vi "Antipinch.vi"(7 "Model Name":T3, 8 "Error In":errorcluster, 9 "Intialize?":bool=TRUE, 10 "Inputs":T1, 11 "Start SM":dbl=20.0 format="%#_13g") -> (0 "error out":errorcluster, 1 "Completed":bool, 3 "Results":cluster{"Pinch Force":dbl}, 4 "Status":cluster{"Status":string, "Elapsed Time":dbl}, 5 "Graph":dbl[][](array[numeric]))   [LabVIEW 2017]
doc: "Changelog:\n\n------------\nv0.1:\n- Bypass sensor 1 for all front\n\nv0.1:\n- Start Travel time taken from when the start moving command is given (previous state)\n- Total travel time is taken until the movement is stopped"
uses:
  controls/Model Name.ctl
  controls/All Inputs.ctl
  controls/SACB DI.ctl
  controls/Antipinch.ctl
  controls/FGV DO.ctl
panel:
  out "x/y":dbl
  in  "minimum change":dbl=2.0 format="%#_13g"
  in  "AutoCommand":u32=50
  in  "Stall Time":u32=200
  out "Waveform Graph":dbl[][](graph)
  in  "Delay (for Rest)":u32=500
  in  "Timeout (ms)":u32=15000
  # "Inputs"
  # "Variables"
  # "Outputs"
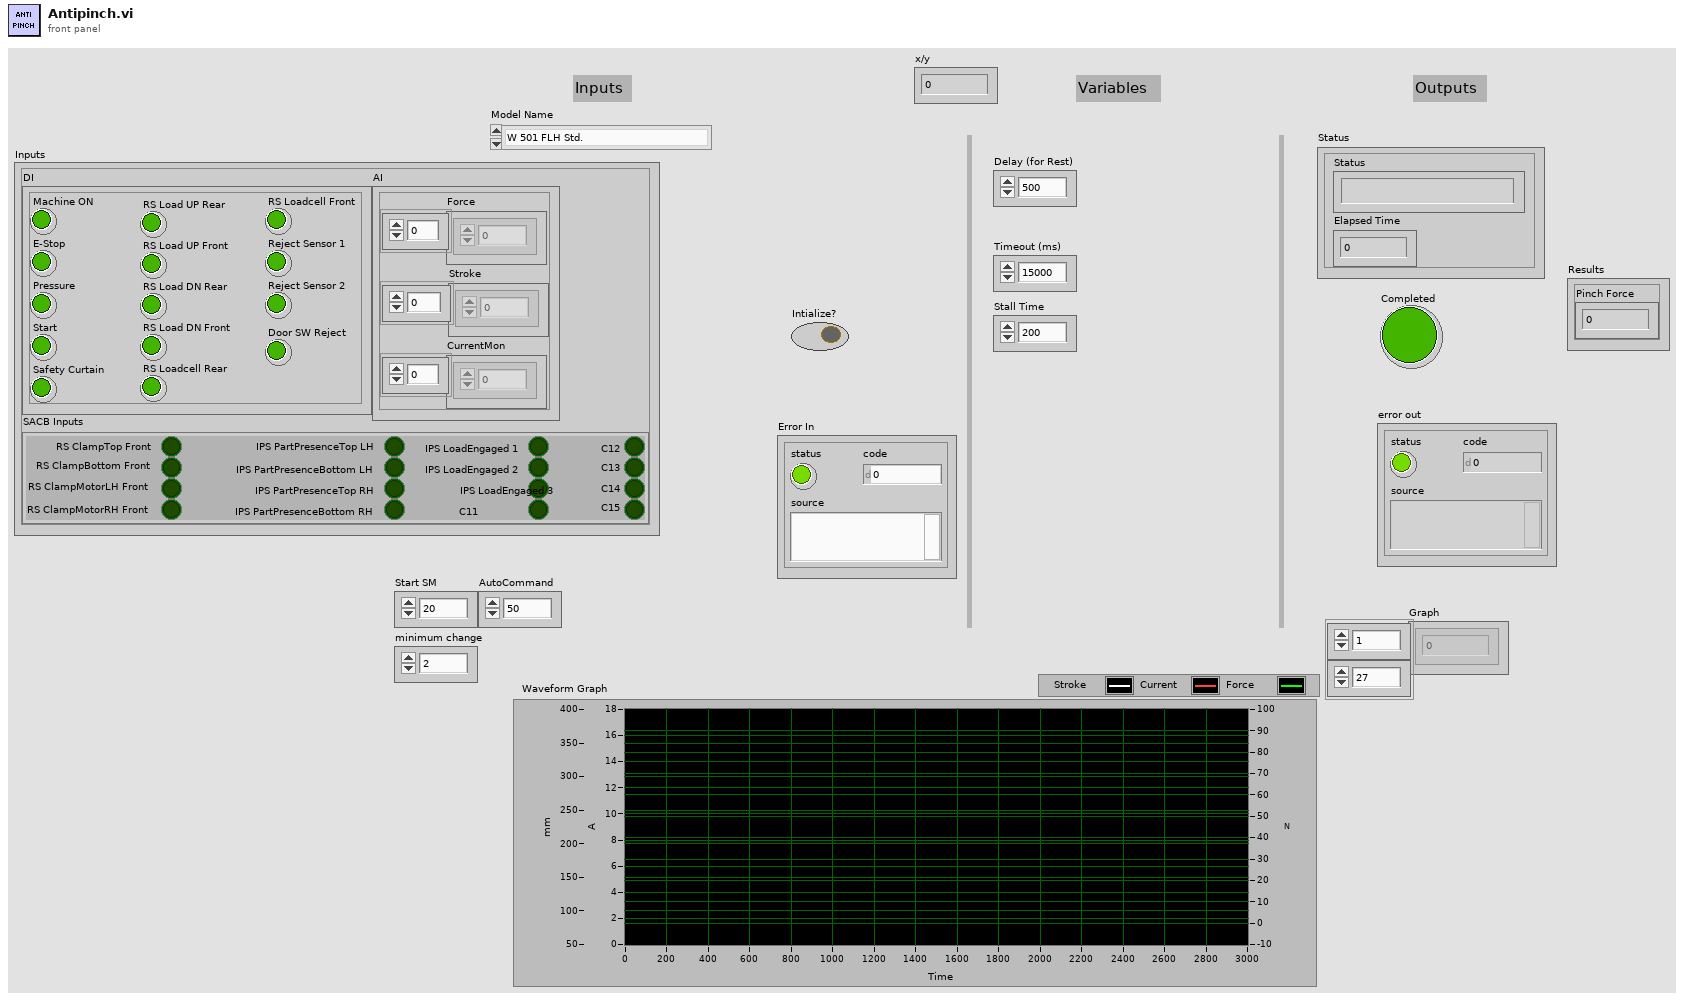
[diagram p1: front panel]
types:
  T1 = typedef "All Inputs.ctl" = cluster{"DI":cluster{"Machine ON":bool, "E-Stop":bool, "Pressure":bool, "Start":bool, "Safety Curtain":bool, "RS Load UP Rear":bool, "RS Load UP Front":bool, "RS Load DN Rear":bool, "RS Load DN Front":bool, "RS Loadcell Rear":bool, "RS Loadcell Front":bool, "Reject Sensor 1":bool, "Reject Sensor 2":bool, "Door SW Reject":bool}, "AI":cluster{"Force":dbl[], "Stroke":dbl[], "CurrentMon":dbl[]}, "SACB Inputs":T2}
  T2 = typedef "SACB DI.ctl" = cluster{"RS ClampTop Front":bool, "RS ClampBottom Front":bool, "RS ClampMotorLH Front":bool, "RS ClampMotorRH Front":bool, "IPS PartPresenceTop LH":bool, "IPS PartPresenceBottom LH":bool, "IPS PartPresenceTop RH":bool, "IPS PartPresenceBottom RH":bool, "IPS LoadEngaged 1":bool, "IPS LoadEngaged 2":bool, "IPS LoadEngaged 3":bool, "C11":bool, "C12":bool, "C13":bool, "C14":bool, "C15":bool}
  T3 = typedef "Model Name.ctl" = enum16{"W 501 FLH Std.", "W 501 FRH Std.", "W 601 FR RH Std", "W 601 FR LH Std", "W 601 RR RH Std", "W 601 RR LH Std", "W 601 FR RH AP", "W 601 FR LH AP", "W 601 RR RH AP", "W 601 RR LH AP"}
  T4 = typedef "Antipinch.ctl" = enum16{"Initialize", "Check Bottom Position", "Auto UP-1", "Auto UP-2", "Loadcell Front", "Wait for Pinch", "Wait for Reversal", "Wait for Stop", "Loadcell Rear & Rest", "Done", "Error"}
  T5 = typedef "FGV DO.ctl" = enum16{"Initialize", "Start Task", "Clamping", "Load CYL", "Contactors", "Loadcell CYL", "BSL", "Read DO", "Clear Tasks", "Clear Task"}
  T6 = typedef "AntiPinch.ctl" = enum16{"Initialize", "Check Bottom Position", "Auto UP-1", "Auto UP-2", "Loadcell Front", "Wait for Pinch", "Wait for Reversal", "Wait for Stop", "Loadcell Rear & Rest", "Done", "Error"}
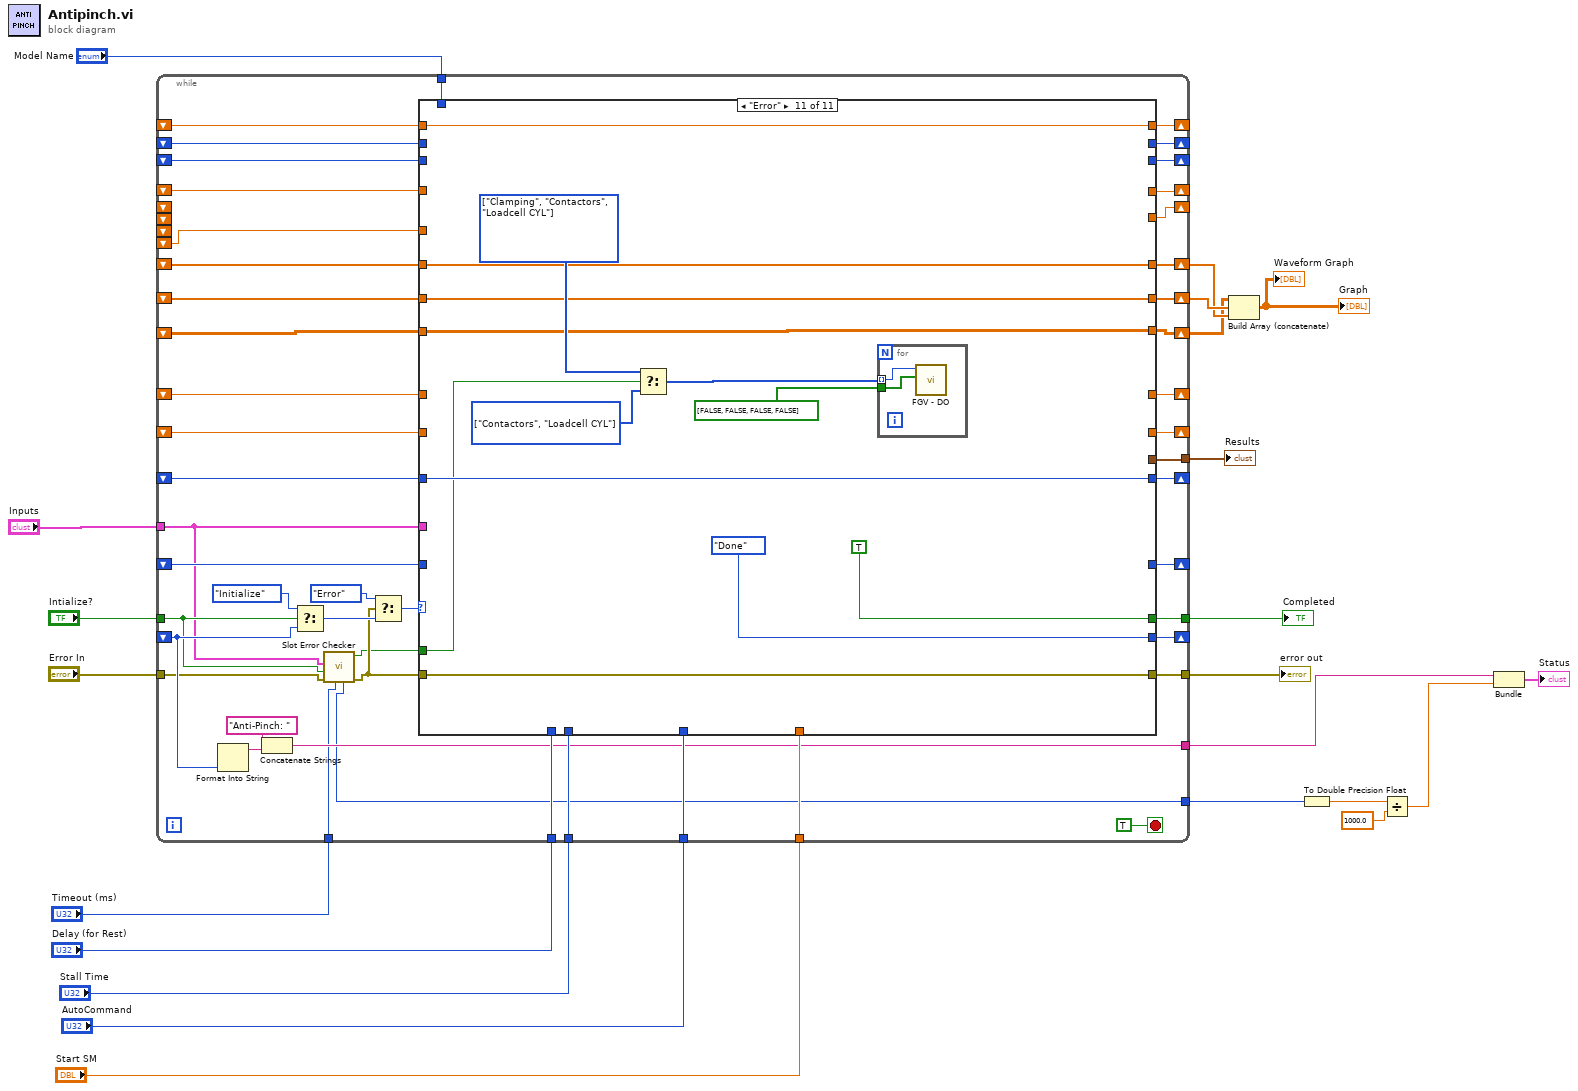
[diagram p0: block diagram]
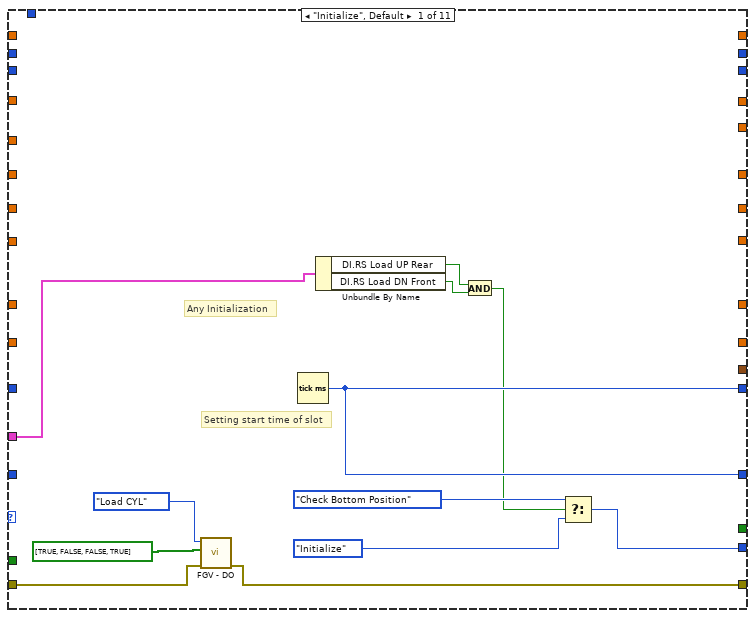
[diagram p2: hidden frame]
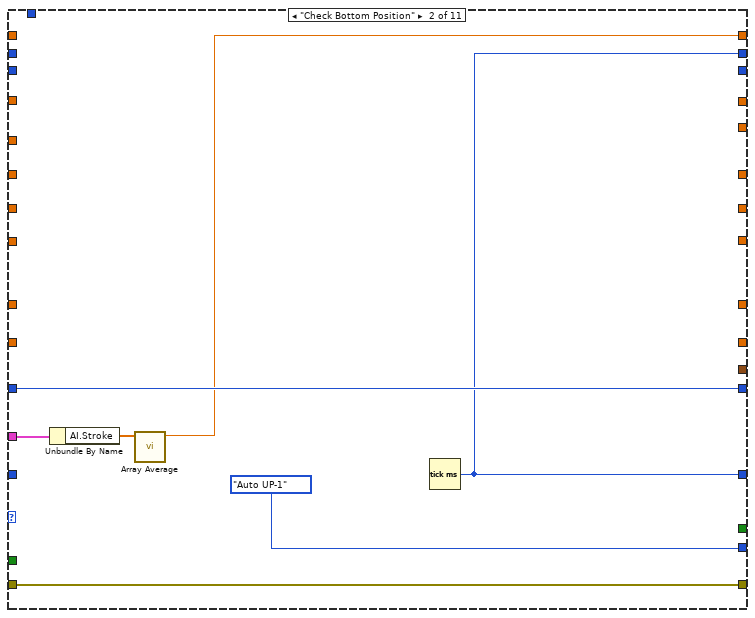
[diagram p3: hidden frame]
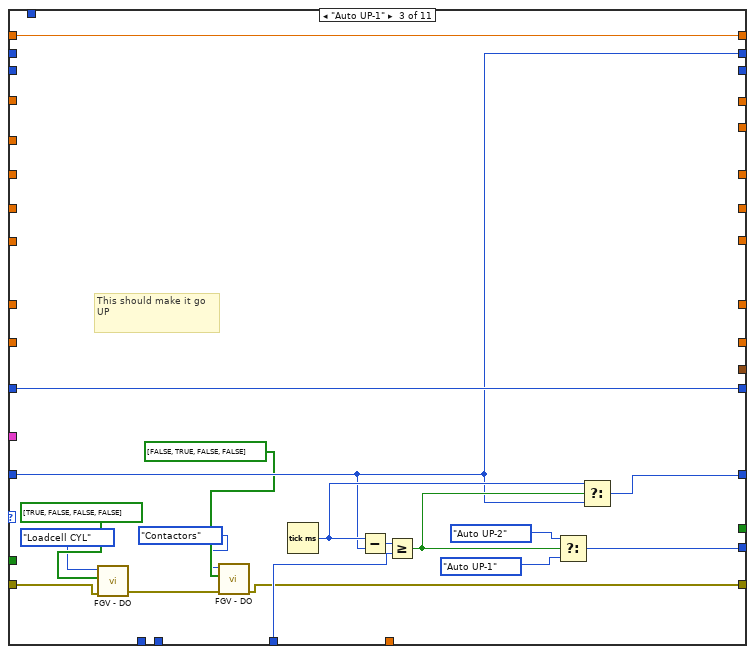
[diagram p4: hidden frame]
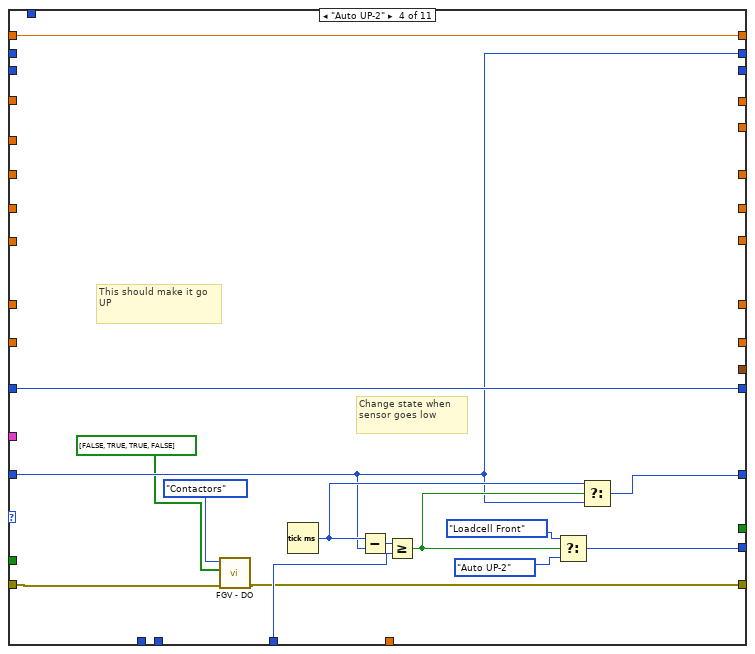
[diagram p5: hidden frame]
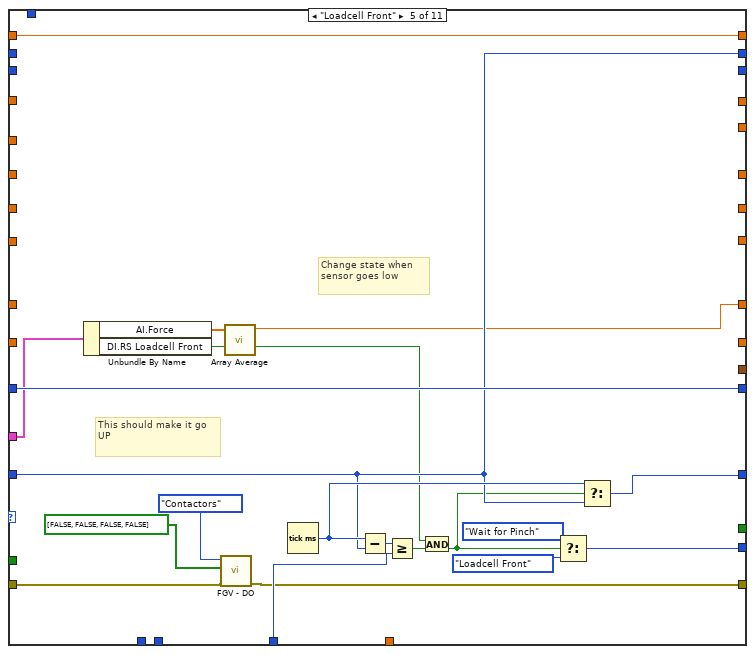
[diagram p6: hidden frame]
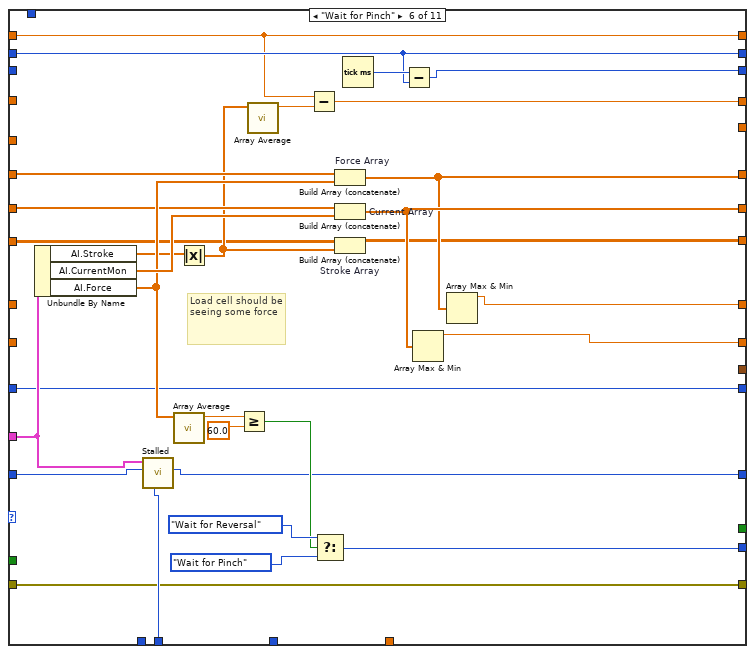
[diagram p7: hidden frame]
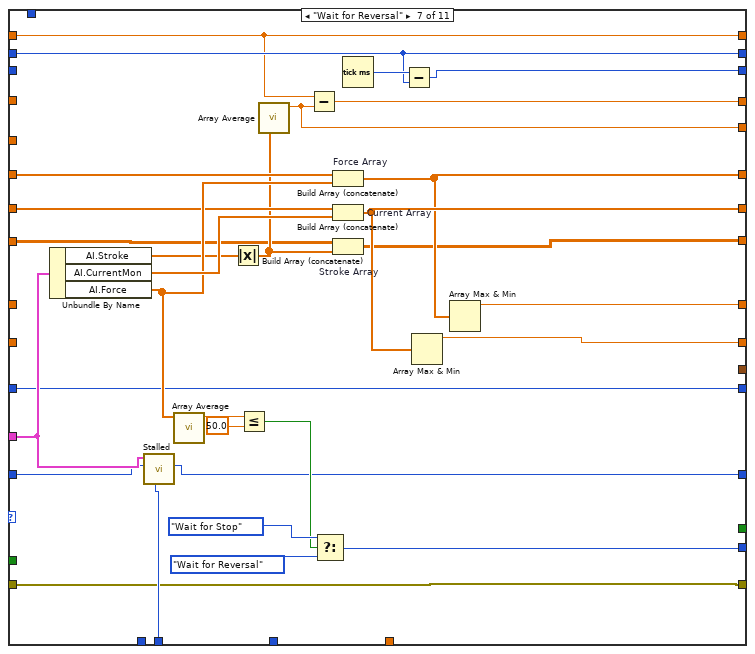
[diagram p8: hidden frame]
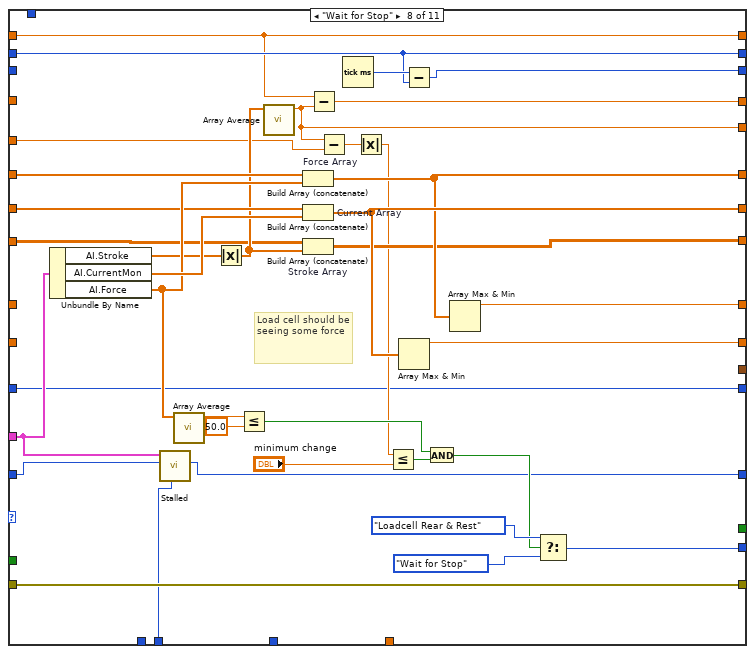
[diagram p9: hidden frame]
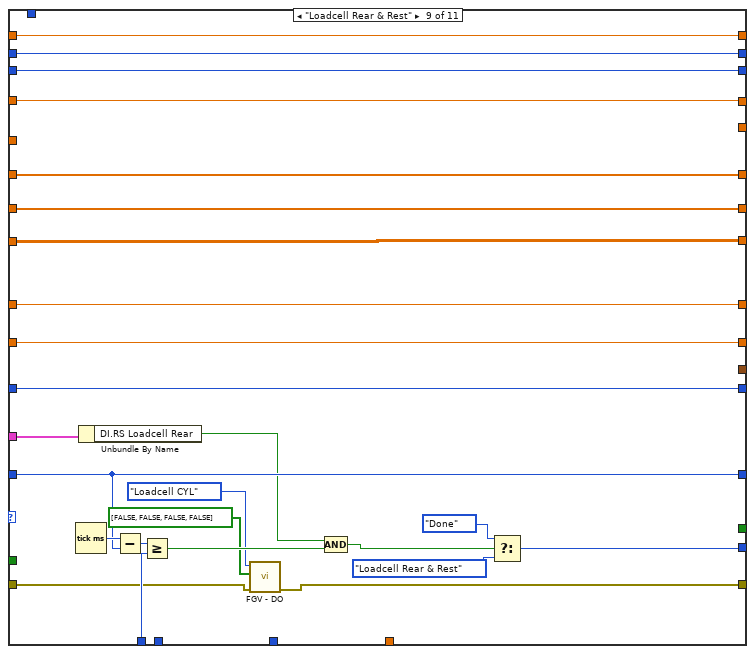
[diagram p10: hidden frame]
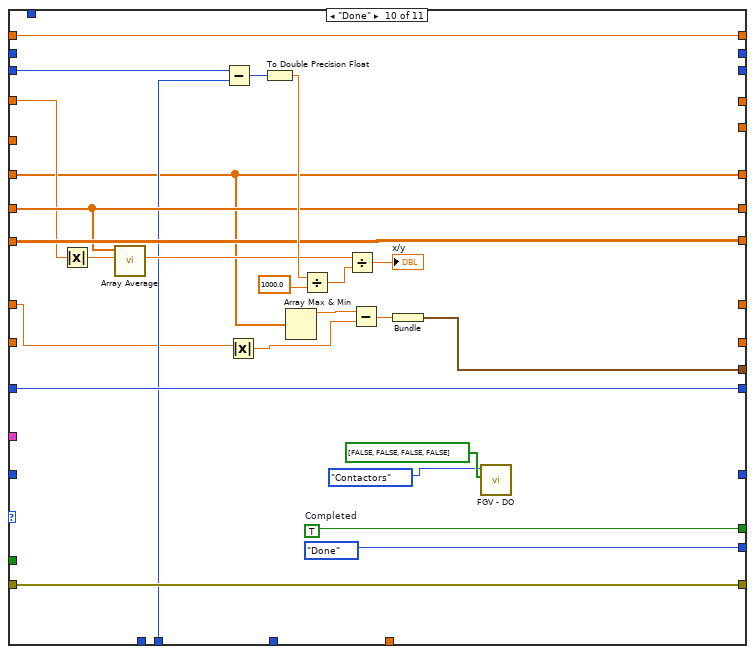
[diagram p11: hidden frame]
diagram:
  n1 = while {
    tunnel: "Intialize?" -> [w30]
    shift-right: [w69] -> _
    shift-left: _ -> [w32]
    shift-right: [w68] -> _
    shift-left: _ -> [w67]
    tunnel: "Error In" -> [w31]
    tunnel: [w66] -> w22
    tunnel: [w65] -> w21
    tunnel: "Inputs" -> [w29]
    tunnel: "Delay (for Rest)" -> [w62]
    tunnel: "Timeout (ms)" -> [w27]
    tunnel: "Model Name" -> [w61]
    shift-right: [w60] -> _
    shift-left: _ -> [w59]
    shift-right: [w58] -> w2
    shift-left: _ -> [w57]
    shift-right: [w56] -> _
    shift-left: _ -> [w55]
    tunnel: [w54] -> w15
    shift-right: [w53] -> _
    shift-left: _ -> [w52]
    tunnel: [w26] -> w10
    shift-right: [w50] -> _
    shift-left: _ -> [w49]
    shift-right: [w48] -> w9
    shift-left: _ -> [w47]
    shift-right: [w46] -> w7
    shift-left: _ -> [w45]
    shift-right: [w44] -> _
    shift-left: _ -> [w43]
    shift-right: [w42] -> _
    shift-left: _ -> [w41]
    tunnel: "Stall Time" -> [w40]
    tunnel: "Start SM" -> [w39]
    tunnel: "AutoCommand" -> [w38]
    shift-right: [w37] -> _
    shift-left: _ -> [_]
    shift-left: _ -> [_]
    shift-left: _ -> [_]
    shift-left: _ -> [w36]
    tunnel: [w33] -> w3
    shift-right: [w24] -> _
    shift-left: _ -> [w23]
    stop <- TRUE stop-if-true
    n2 = Format Into String(w32) -> (resulting string=w35:string)  [unwired: 3 in, 1 out]
    n3 = Concatenate Strings("Anti-Pinch: ", w35) -> (w33:string)
    n4 = Select(t=Antipinch."Initialize", s=w30, f=w32) -> (s? t:f=w64:T4)
    n5 = call "Slot Error Checker.vi"("Timeout (ms)"=w27, "error in (no error)"=w31, "Intialize?"=w30, "Inputs"=w29) -> ("error out"=w28:errorcluster, "Safety Interrupt?"=w25:bool, "Slot Time"=w26:u32)  [unwired: 5 in]
    n6 = Select(t=Antipinch."Error", s=w28, f=w64) -> (s? t:f=w51:T4)
    n7 = case shown="\"Error\"" w51 {
      tunnel: [w81 AntiPinch."Auto UP-1" w104 w119 w139 w171 w201 w237 w261 Antipinch."Done" Antipinch."Done"] -> w69
      tunnel: [w83 w84 w99 w114 w134 w149 w178 w207 w263 _ _] -> w68
      tunnel: w67 -> [_ _ w100 w115 w135 w150 w179 w209 w263 _ _]
      tunnel: w28 -> [w73 w89 w96 w110 w125 w146 w175 w220 w241 w287 w301]
      tunnel: [w72 w89 w92 w109 w124 w146 w175 w220 w240 w287 w301] -> w66
      tunnel: [_ _ _ _ _ _ _ _ _ w286 TRUE ("Completed")] -> w65
      tunnel: w29 -> [w79 w86 _ _ w132 w145 w180 w205 w244 _ _]
      tunnel: [w83 w90 w108 w123 w143 w144 w174 w204 w257 w285 w298] -> w24
      tunnel: w23 -> [_ w90 w108 w123 w143 w144 w174 w204 w257 w285 w298]
      tunnel: w62 -> [_ _ _ _ _ _ _ _ w256 _ _]
      tunnel: w61 -> [_ _ _ _ _ _ _ _ _ _ _]
      tunnel: [_ w84 w100 w115 w135 w163 w193 w229 w253 _ _] -> w60
      tunnel: w59 -> [_ _ _ _ _ w163 w193 w229 w253 _ _]
      tunnel: [_ _ _ _ _ w164 w194 w230 w255 w280 w291] -> w58
      tunnel: w57 -> [_ _ _ _ _ w151 w181 w210 w255 w280 w291]
      tunnel: [_ _ _ _ _ w165 w195 w231 w254 _ _] -> w56
      tunnel: w55 -> [_ _ _ _ _ _ _ _ w254 w276 _]
      tunnel: [_ _ _ _ _ _ _ _ _ w281 _] -> w54
      tunnel: [_ _ _ _ _ w169 w199 w235 w252 _ _] -> w53
      tunnel: w52 -> [_ _ _ _ _ _ _ _ w252 _ _]
      tunnel: [_ w85 w107 w122 w142 w155 w185 w221 w251 w277 w297] -> w50
      tunnel: w49 -> [_ _ w107 w122 w142 w155 w185 w221 w251 w277 w297]
      tunnel: [_ _ _ _ _ w167 w197 w233 w248 w279 w290] -> w48
      tunnel: w47 -> [_ _ _ _ _ w159 w189 w225 w248 w279 w290]
      tunnel: [_ _ _ _ _ w166 w196 w232 w249 w272 w289] -> w46
      tunnel: w45 -> [_ _ _ _ _ w158 w188 w224 w249 w272 w289]
      tunnel: [_ _ _ _ w128 w147 w176 w206 w247 _ _] -> w44
      tunnel: w43 -> [_ _ _ _ _ _ _ _ w247 w271 _]
      tunnel: [_ _ _ _ _ w153 w184 w218 w250 _ _] -> w42
      tunnel: w41 -> [_ _ _ _ _ _ _ _ w250 w273 _]
      tunnel: w40 -> [_ _ _ _ _ w148 w177 w208 _ w274 _]
      tunnel: w25 -> [_ _ _ _ _ _ _ _ _ _ w292]
      tunnel: w39 -> [_ _ _ _ _ _ _ _ _ _ _]
      tunnel: w38 -> [_ _ w103 w118 w138 _ _ _ _ _ _]
      tunnel: [_ _ _ _ _ _ w182 w217 _ _ _] -> w37
      tunnel: w36 -> [_ _ _ _ _ _ _ w216 _ _ _]
      frame "Initialize", Default {
        # "Setting start time of slot"
        # "Any Initialization"
        n8 = call "FGV - DO.vi"("error in"=w73, "Digital Outs"=bool[] [TRUE, FALSE, FALSE, TRUE], "State"=FGV_DO."Load CYL") -> ("error out"=w72:errorcluster)  [unwired: 7 in, 1 out]
        n9 = Tick Count (ms)() -> (millisecond timer value=w83:u32)
        n10 = Unbundle By Name(w79) -> ("DI.RS Load UP Rear"=w78:bool, "DI.RS Load DN Front"=w77:bool)
        n11 = And(x=w78, y=w77) -> (x .and. y?=w76:bool)
        n12 = Select(t=Antipinch."Check Bottom Position", s=w76, f=Antipinch."Initialize") -> (s? t:f=w81:T4)
      }
      frame "Check Bottom Position" {
        n13 = Unbundle By Name(w86) -> ("AI.Stroke"=w87:dbl[])
        n14 = call "Array Average.vi"("data"=w87) -> ("Numeric"=w85:dbl)  [unwired: 10 in]
        n15 = Tick Count (ms)() -> (millisecond timer value=w84:u32)
      }
      frame "Auto UP-1" {
        # "This should make it go UP"
        n16 = call "FGV - DO.vi"("error in"=w96, "Digital Outs"=bool[] [TRUE, FALSE, FALSE, FALSE], "State"=FGV_DO."Loadcell CYL") -> ("error out"=w93:errorcluster)  [unwired: 7 in, 1 out]
        n17 = call "FGV - DO.vi"("error in"=w93, "Digital Outs"=bool[] [FALSE, TRUE, FALSE, FALSE], "State"=FGV_DO."Contactors") -> ("error out"=w92:errorcluster)  [unwired: 7 in, 1 out]
        n18 = Tick Count (ms)() -> (millisecond timer value=w101:u32)
        n19 = Subtract(x=w101, y=w100) -> (x-y=w106:u32)
        n20 = Greater Or Equal?(x=w106, y=w103) -> (x >= y?=w102:bool)
        n21 = Select(t=AntiPinch."Auto UP-2", s=w102, f=AntiPinch."Auto UP-1") -> (s? t:f=w104:T6)
        n22 = Select(t=w101, s=w102, f=w100) -> (s? t:f=w99:u32)
      }
      frame "Auto UP-2" {
        # "Change state when sensor goes low"
        # "This should make it go UP"
        n23 = call "FGV - DO.vi"("error in"=w110, "Digital Outs"=bool[] [FALSE, TRUE, TRUE, FALSE], "State"=FGV_DO."Contactors") -> ("error out"=w109:errorcluster)  [unwired: 7 in, 1 out]
        n24 = Tick Count (ms)() -> (millisecond timer value=w116:u32)
        n25 = Subtract(x=w116, y=w115) -> (x-y=w121:u32)
        n26 = Greater Or Equal?(x=w121, y=w118) -> (x >= y?=w117:bool)
        n27 = Select(t=AntiPinch."Loadcell Front", s=w117, f=AntiPinch."Auto UP-2") -> (s? t:f=w119:T6)
        n28 = Select(t=w116, s=w117, f=w115) -> (s? t:f=w114:u32)
      }
      frame "Loadcell Front" {
        # "Change state when sensor goes low"
        # "This should make it go UP"
        n29 = Unbundle By Name(w132) -> ("AI.Force"=w129:dbl[], "DI.RS Loadcell Front"=w130:bool)
        n30 = call "FGV - DO.vi"("error in"=w125, "Digital Outs"=bool[] [FALSE, FALSE, FALSE, FALSE], "State"=FGV_DO."Contactors") -> ("error out"=w124:errorcluster)  [unwired: 7 in, 1 out]
        n31 = call "Array Average.vi"("data"=w129) -> ("Numeric"=w128:dbl)  [unwired: 10 in]
        n32 = Tick Count (ms)() -> (millisecond timer value=w136:u32)
        n33 = Subtract(x=w136, y=w135) -> (x-y=w141:u32)
        n34 = Greater Or Equal?(x=w141, y=w138) -> (x >= y?=w137:bool)
        n35 = And(x=w130, y=w137) -> (x .and. y?=w131:bool)
        n36 = Select(t=AntiPinch."Wait for Pinch", s=w131, f=AntiPinch."Loadcell Front") -> (s? t:f=w139:T6)
        n37 = Select(t=w136, s=w131, f=w135) -> (s? t:f=w134:u32)
      }
      frame "Wait for Pinch" {
        # "Load cell should be seeing some force"
        n38 = Unbundle By Name(w145) -> ("AI.Stroke"=w157:dbl[], "AI.CurrentMon"=w168:dbl[], "AI.Force"=w161:dbl[])
        n39 = call "Stalled.vi"("Stall Time (ms)"=w148, "millisecond timer value in"=w150, "Inputs"=w145) -> ("millisecond timer value out"=w149:u32)  [unwired: 7 in, 1 out]
        n40 = call "Array Average.vi"("data"=w161) -> ("Numeric"=w160:dbl)  [unwired: 10 in]
        n41 = Absolute Value(x=w157) -> (abs(x)=w156:dbl[])
        n42 = Greater Or Equal?(x=w160, y=60.0) -> (x >= y?=w152:bool)
        n43 = call "Array Average.vi"("data"=w156) -> ("Numeric"=w154:dbl)  [unwired: 10 in]
        n44 = Subtract(x=w155, y=w154) -> (x-y=w153:dbl)
        n45 = Select(t=AntiPinch."Wait for Reversal", s=w152, f=AntiPinch."Wait for Pinch") -> (s? t:f=w171:T6)
        n46 = Build Array (concatenate) "Force Array"(w158, w161) -> (w166:dbl[])
        n47 = Build Array (concatenate) "Current Array"(w159, w168) -> (w167:dbl[])
        n48 = Build Array (concatenate) "Stroke Array"(w151, w156) -> (w164:dbl[][])
        n49 = Tick Count (ms)() -> (millisecond timer value=w170:u32)
        n50 = Subtract(x=w170, y=w163) -> (x-y=w165:u32)
        n51 = Array Max & Min(array=w167) -> (max value=w169:dbl)  [unwired: 3 out]
        n52 = Array Max & Min(array=w166) -> (max value=w147:dbl)  [unwired: 3 out]
      }
      frame "Wait for Reversal" {
        n53 = Unbundle By Name(w180) -> ("AI.Stroke"=w187:dbl[], "AI.CurrentMon"=w198:dbl[], "AI.Force"=w191:dbl[])
        n54 = call "Stalled.vi"("Stall Time (ms)"=w177, "millisecond timer value in"=w179, "Inputs"=w180) -> ("millisecond timer value out"=w178:u32)  [unwired: 7 in, 1 out]
        n55 = call "Array Average.vi"("data"=w191) -> ("Numeric"=w190:dbl)  [unwired: 10 in]
        n56 = Absolute Value(x=w187) -> (abs(x)=w186:dbl[])
        n57 = Less Or Equal?(x=w190, y=50.0) -> (x <= y?=w183:bool)
        n58 = call "Array Average.vi"("data"=w186) -> ("Numeric"=w182:dbl)  [unwired: 10 in]
        n59 = Subtract(x=w185, y=w182) -> (x-y=w184:dbl)
        n60 = Select(t=AntiPinch."Wait for Stop", s=w183, f=AntiPinch."Wait for Reversal") -> (s? t:f=w201:T6)
        n61 = Build Array (concatenate) "Force Array"(w188, w191) -> (w196:dbl[])
        n62 = Build Array (concatenate) "Current Array"(w189, w198) -> (w197:dbl[])
        n63 = Build Array (concatenate) "Stroke Array"(w181, w186) -> (w194:dbl[][])
        n64 = Tick Count (ms)() -> (millisecond timer value=w200:u32)
        n65 = Subtract(x=w200, y=w193) -> (x-y=w195:u32)
        n66 = Array Max & Min(array=w197) -> (max value=w199:dbl)  [unwired: 3 out]
        n67 = Array Max & Min(array=w196) -> (max value=w176:dbl)  [unwired: 3 out]
      }
      frame "Wait for Stop" {
        # "Load cell should be seeing some force"
        n68 = Unbundle By Name(w205) -> ("AI.Stroke"=w223:dbl[], "AI.CurrentMon"=w234:dbl[], "AI.Force"=w227:dbl[])
        n69 = call "Stalled.vi"("Stall Time (ms)"=w208, "millisecond timer value in"=w209, "Inputs"=w205) -> ("millisecond timer value out"=w207:u32)  [unwired: 7 in, 1 out]
        n70 = call "Array Average.vi"("data"=w227) -> ("Numeric"=w226:dbl)  [unwired: 10 in]
        n71 = Absolute Value(x=w223) -> (abs(x)=w222:dbl[])
        n72 = Less Or Equal?(x=w226, y=50.0) -> (x <= y?=w219:bool)
        n73 = call "Array Average.vi"("data"=w222) -> ("Numeric"=w217:dbl)  [unwired: 10 in]
        n74 = Build Array (concatenate) "Force Array"(w224, w227) -> (w232:dbl[])
        n75 = Build Array (concatenate) "Current Array"(w225, w234) -> (w233:dbl[])
        n76 = Build Array (concatenate) "Stroke Array"(w210, w222) -> (w230:dbl[][])
        n77 = Subtract(x=w221, y=w217) -> (x-y=w218:dbl)
        n78 = Subtract(x=w217, y=w216) -> (x-y=w215:dbl)
        n79 = Tick Count (ms)() -> (millisecond timer value=w236:u32)
        n80 = Absolute Value(x=w215) -> (abs(x)=w214:dbl)
        n81 = Less Or Equal?(x=w214, y="minimum change") -> (x <= y?=w211:bool)
        n82 = Array Max & Min(array=w233) -> (max value=w235:dbl)  [unwired: 3 out]
        n83 = Subtract(x=w236, y=w229) -> (x-y=w231:u32)
        n84 = And(x=w219, y=w211) -> (x .and. y?=w212:bool)
        n85 = Array Max & Min(array=w232) -> (max value=w206:dbl)  [unwired: 3 out]
        n86 = Select(t=AntiPinch."Loadcell Rear & Rest", s=w212, f=AntiPinch."Wait for Stop") -> (s? t:f=w237:T6)
      }
      frame "Loadcell Rear & Rest" {
        n87 = Tick Count (ms)() -> (millisecond timer value=w264:u32)
        n88 = Unbundle By Name(w244) -> ("DI.RS Loadcell Rear"=w246:bool)
        n89 = Subtract(x=w264, y=w263) -> (x-y=w262:u32)
        n90 = Greater Or Equal?(x=w262, y=w256) -> (x >= y?=w260:bool)
        n91 = call "FGV - DO.vi"("error in"=w241, "Digital Outs"=bool[] [FALSE, FALSE, FALSE, FALSE], "State"=FGV_DO."Loadcell CYL") -> ("error out"=w240:errorcluster)  [unwired: 7 in, 1 out]
        n92 = Compound Arithmetic op=AND(w246, w260) -> (w245:bool)
        n93 = Select(t=Antipinch."Done", s=w245, f=Antipinch."Loadcell Rear & Rest") -> (s? t:f=w261:T4)
      }
      frame "Done" {
        w286 = TRUE  # Completed
        n94 = Absolute Value(x=w273) -> (abs(x)=w278:dbl)
        n95 = call "Array Average.vi"("data"=w279) -> ()  [unwired: 10 in, 1 out]
        n96 = Subtract(x=w276, y=w274) -> (x-y=w275:u32)
        n97 = Absolute Value(x=w271) -> (abs(x)=w270:dbl)
        n98 = To Double Precision Float(number=w275) -> (double precision float=w283:dbl)
        n99 = Array Max & Min(array=w272) -> (max value=w269:dbl)  [unwired: 3 out]
        n100 = Divide(x=w283, y=1000.0) -> (x/y=w282:dbl)
        n101 = Divide(x=w278, y=w282) -> (x/y=→"x/y":dbl)
        n102 = Subtract(x=w269, y=w270) -> (x-y=w268:dbl)
        n103 = Bundle(w268) -> (w281:cluster{dbl})  [unwired: 1 in]
        n104 = call "FGV - DO.vi"("Digital Outs"=bool[] [FALSE, FALSE, FALSE, FALSE], "State"=FGV_DO."Contactors") -> ()  [unwired: 8 in, 2 out]
      }
      frame "Error" {
        w293 = T5[] [enum."Contactors", enum."Loadcell CYL"] items=["Initialize", "Start Task", "Clamping", "Load CYL", "Contactors", "Loadcell CYL", "BSL", "Read DO", "Clear Tasks", "Clear Task"]
        w295 = T5[] [enum."Clamping", enum."Contactors", enum."Loadcell CYL"] items=["Initialize", "Start Task", "Clamping", "Load CYL", "Contactors", "Loadcell CYL", "BSL", "Read DO", "Clear Tasks", "Clear Task"]
        n105 = Select(t=w295, s=w292, f=w293) -> (s? t:f=w294:T5[])
        n106 = for {
          tunnel: w294 -> [w303] mode=indexing
          tunnel: bool[] [FALSE, FALSE, FALSE, FALSE] ("Digital Outs") -> [w302]
          n107 = call "FGV - DO.vi"("Digital Outs"=w302, "State"=w303) -> ()  [unwired: 8 in, 2 out]
        }
      }
    }
  }
  "error out" <- w22
  "Completed" <- w21
  "Results" <- w15
  n108 = Build Array (concatenate)(w2, w9, w7) -> (→"Graph" →"Waveform Graph":dbl[][])
  n109 = To Double Precision Float(number=w10) -> (double precision float=w14:dbl)
  n110 = Divide(x=w14, y=1000.0) -> (x/y=w12:dbl)
  n111 = Bundle(w3, w12) -> (→"Status":cluster{string, dbl})  [unwired: 1 in]
